vi "Create Policy.vi"(6 "Path":string="/", 7 "Description":string, 8 "error in (no error)":errorcluster, 9 "Document":string, 10 "Name":string, 11 "IAM Session in":refnum<class "IAM Session.lvclass">) -> (0 "error out":errorcluster, 2 "Created Policy":T1, 3 "IAM Session out":refnum<class "IAM Session.lvclass">)   [LabVIEW 2015, in "NI_AWS_IAM.lvlib" / "IAM Session.lvclass"]
uses:
  IAM Session.lvclass
  Policy.ctl
  Core/HTTP Request/Request Options.ctl
  Core/HTTP Request/Name Value Pair.ctl
  Core/HTTP Request/Region handling.ctl
  Core/HTTP Request/URL formatting.ctl
  Core/HTTP Request/HTTP Request.lvclass
  NI_AWS_IAM.lvlib
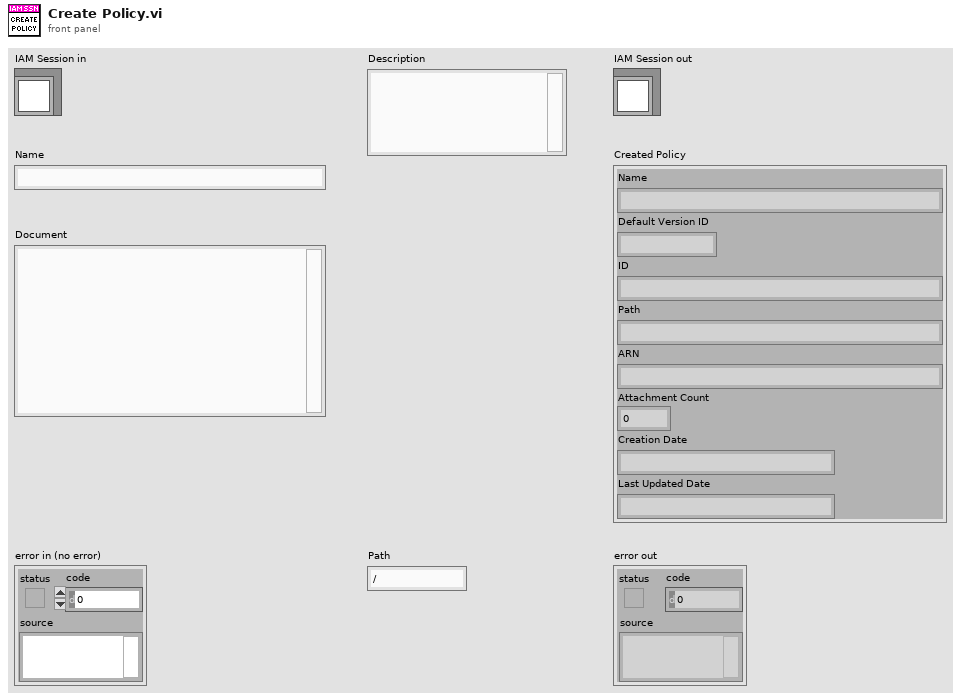
[diagram p1: front panel]
types:
  T1 = typedef "NI_AWS_IAM.lvlib/Policy.ctl" = cluster{"Name":string, "Default Version ID":string, "ID":string, "Path":string, "ARN":string, "Attachment Count":i32, "Creation Date":string, "Last Updated Date":string}
  T2 = typedef "NI_AWS_Core.lvlib/HTTP Request.lvclass/Name Value Pair.ctl" = cluster{"name":string, "value":string}
  T3 = typedef "NI_AWS_Core.lvlib/HTTP Request.lvclass/Request Options.ctl" = cluster{"request headers":T2[], "request parameters":T2[], "request body":string, "region handling":T4, "URL formatting":T5}
  T4 = typedef "NI_AWS_Core.lvlib/HTTP Request.lvclass/Region handling.ctl" = enum16{"use region everywhere", "use region (authentication only)", "use region (URL only)", "ignore region everwhere"}
  T5 = typedef "NI_AWS_Core.lvlib/HTTP Request.lvclass/URL formatting.ctl" = enum16{"region-", "region."}
  T6 = typedef "NI_AWS_Core.lvlib/HTTP Request.lvclass/Response.ctl" = cluster{"Headers":string, "Body":string}
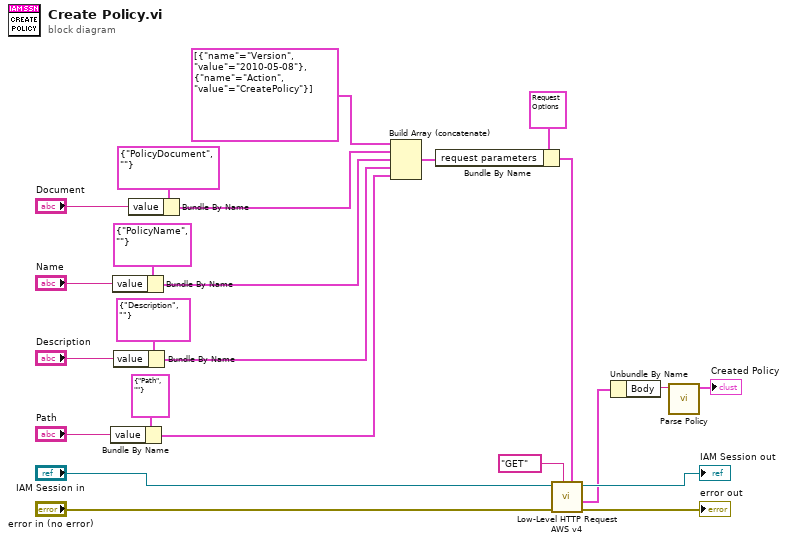
[diagram p0: block diagram]
diagram:
  n1 = Bundle By Name(cluster=T2 {"name"="Path", "value"=""} ("Name Value Pair"), "value"="Path") -> (w4:T2)
  n2 = Bundle By Name(cluster=T2 {"name"="PolicyName", "value"=""} ("Name Value Pair"), "value"="Name") -> (w10:T2)
  n3 = Bundle By Name(cluster=T2 {"name"="Description", "value"=""} ("Name Value Pair"), "value"="Description") -> (w7:T2)
  n4 = Bundle By Name(cluster=T2 {"name"="PolicyDocument", "value"=""} ("Name Value Pair"), "value"="Document") -> (w11:T2)
  n5 = Build Array (concatenate)(T2[] [{"name"="Version", "value"="2010-05-08"}, {"name"="Action", "value"="CreatePolicy"}], w11, w10, w7, w4) -> (w16:T2[])
  n6 = Bundle By Name(cluster=T3 {"request headers"=[], "request parameters"=[], "request body"="", "region handling"=enum."use region everywhere", "URL formatting"=enum."region."} ("Request Options"), "request parameters"=w16) -> (w18:T3)
  n7 = call "Low-Level HTTP Request AWS v4.vi"("Request Options"=w18, "HTTP-Verb"="GET", "error in (no error)"="error in (no error)", "AWS Core in"="IAM Session in") -> ("error out"=→"error out":errorcluster, "Response"=w1:T6, "AWS Core out"=→"IAM Session out":refnum<class "IAM Session.lvclass">)  [unwired: 4 in, 1 out]
  n8 = Unbundle By Name(w1) -> ("Body"=w2:string)
  n9 = call "Parse Policy.vi"("Response body"=w2) -> ("Policy"=→"Created Policy":T1)  [unwired: 10 in]
